vi "HW_Poll_Tracker_1x.vi"(8 "error in":errorcluster, 11 "VISA resource name in":refnum<visa-resource-name>="ASRL3::INSTR") -> (0 "error out":errorcluster, 1 "Read buffer":string, 2 "Parameters output":T1, 3 "VISA resource name out":refnum<visa-resource-name>)   [LabVIEW 2018]
panel:
  out "Sensors response":string
  out "Port data status":i32
  out "Port data status index":i32
  out "FPS status":i32
  out "Poll records":u32
  out "FPS target index":i32
  out "Matrix mode status":string
  out "Matrix mode index":i32
  out "Coordinate mode status":string
  out "Coordinate mode index":i32
  out "Binary mode status":string
  out "Binary mode index":i32
  out "Array of tokens":string[](array[string])
  out "token index":i32
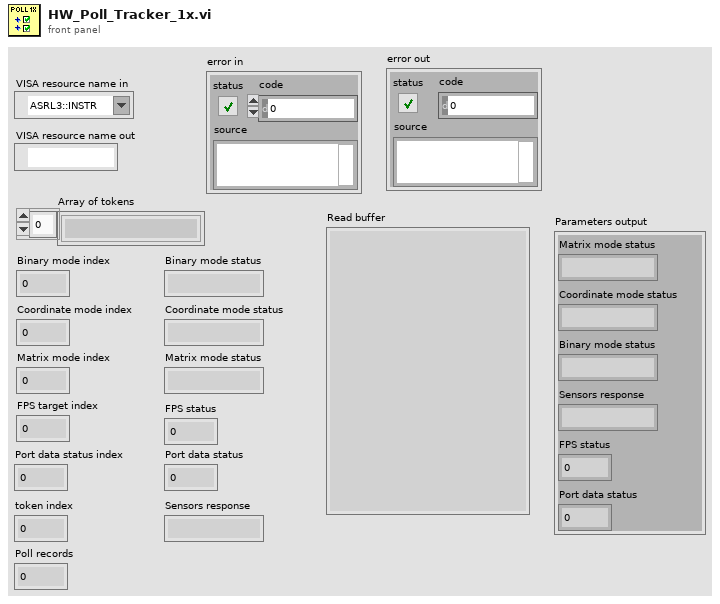
[diagram p1: front panel]
types:
  T1 = cluster{"Matrix mode status":string, "Coordinate mode status":string, "Binary mode status":string, "Sensors response":string, "FPS status":i32, "Port data status":i32}
  T2 = cluster{"token string":string, "token string":string, "token string":string, "trimmed string":string, i32, i32}
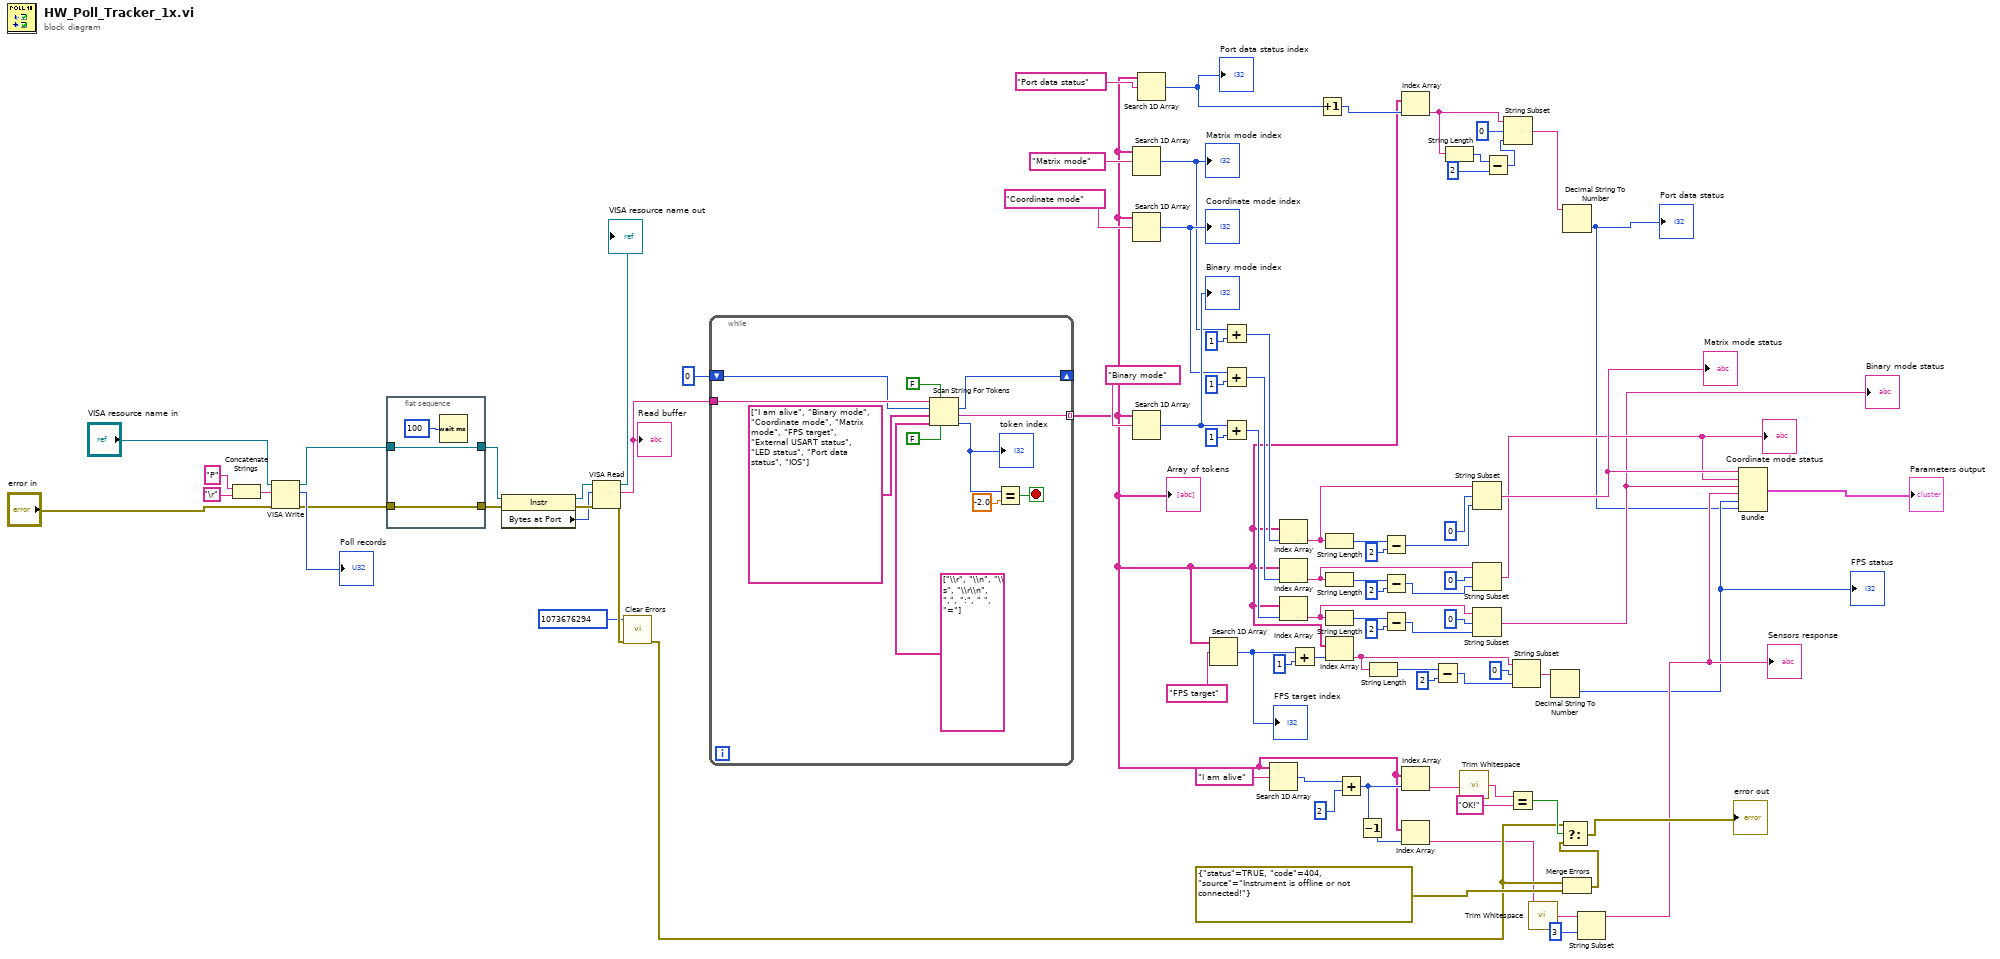
[diagram p0: block diagram]
diagram:
  n1 = Concatenate Strings("P" ("write buffer"), "\r") -> (w86:string)
  n2 = VISA Write(VISA resource name="VISA resource name in", write buffer=w86, error in (no error)="error in") -> (VISA resource name out=w62:refnum<visa-resource-name>, return count=→"Poll records":u32, error out=w60:errorcluster)
  n3 = flat-sequence {
    tunnel: [w90] -> w63
    tunnel: w62 -> [w90]
    tunnel: [w89] -> w61
    tunnel: w60 -> [w89]
    frame #0 {
      n4 = Wait (ms)(milliseconds to wait=u32 100) -> ()  [unwired: 1 out]
    }
  }
  n5 = property class="Instr"(reference=w63, error in=w61) -> (reference out=w84:refnum<visa-resource-name>, error out=w83:errorcluster, "Bytes at Port"=w82:u32)
  n6 = VISA Read(VISA resource name=w84, byte count=w82, error in (no error)=w83) -> (VISA resource name out=→"VISA resource name out":refnum<visa-resource-name>, read buffer=w81:string, error out=w18:errorcluster)  [unwired: 1 out]
  "Read buffer" <- w81
  n7 = call <vilib>:"Clear Errors.vi"("error in (no error)"=w18, "specific error code to clear (0: all)"=1073676294) -> ("error out"=w17:errorcluster)  [unwired: 4 in, 1 out]
  n8 = while {
    tunnel: w81 -> [w102]
    tunnel: [w94] -> w14 mode=indexing
    shift-right: [w93] -> _
    shift-left: 0 ("offset past token") -> [w92]
    stop <- w100 stop-if-true
    n9 = Scan String For Tokens(4:FALSE ("use cached delim/oper data? (F)"), 5:FALSE ("allow empty tokens? (F)"), 6:string[] ["\\r", "\\n", "\\s", "\\r\\n", ",", ":", " ", "="] ("delimiters"), 7:string[] ["I am alive", "Binary mode", "Coordinate mode", "Matrix mode", "FPS target", "External USART status", "LED status", "Port data status", "IOS"] ("Tokens"), 8:w92, 9:w102) -> (0:w98:i32, 1:w94:string, 2:w93:i32)  [unwired: 1 out]
    "token index" <- w98
    n10 = Equal?(x=w98, y=-2.0) -> (x = y?=w100:bool)
  }
  "Array of tokens" <- w14
  n11 = Search 1D Array(1D array=w14, element="Matrix mode") -> (index of element=w70:i32)  [unwired: 1 in]
  "Matrix mode index" <- w70
  n12 = Search 1D Array(1D array=w14, element="Coordinate mode") -> (index of element=w74:i32)  [unwired: 1 in]
  "Coordinate mode index" <- w74
  n13 = Search 1D Array(1D array=w14, element="Binary mode") -> (index of element=w78:i32)  [unwired: 1 in]
  "Binary mode index" <- w78
  n14 = Search 1D Array(1D array=w14, element="Port data status") -> (index of element=w36:i32)  [unwired: 1 in]
  "Port data status index" <- w36
  n15 = Search 1D Array(1D array=w14, element="FPS target") -> (index of element=w66:i32)  [unwired: 1 in]
  "FPS target index" <- w66
  n16 = Add(x=w70, y=1) -> (x+y=w71:i32)
  n17 = Add(x=w74, y=1) -> (x+y=w75:i32)
  n18 = Add(x=w78, y=1) -> (x+y=w79:i32)
  n19 = Search 1D Array(1D array=w14, element="I am alive") -> (index of element=w27:i32)  [unwired: 1 in]
  n20 = Index Array(array=w14, index=w71) -> (element=w40:string)
  n21 = Index Array(array=w14, index=w75) -> (element=w38:string)
  n22 = Index Array(array=w14, index=w79) -> (element=w57:string)
  n23 = Add(x=w66, y=1) -> (x+y=w67:i32)
  n24 = Increment(x=w36) -> (x+1=w35:i32)
  n25 = String Length(string=w40) -> (length=w52:i32)
  n26 = String Length(string=w38) -> (length=w43:i32)
  n27 = String Length(string=w57) -> (length=w56:i32)
  n28 = Index Array(array=w14, index=w67) -> (element=w39:string)
  n29 = Add(x=w27, y=2) -> (x+y=w15:i32)
  n30 = Decrement(x=w15) -> (x-1=w13:i32)
  n31 = String Length(string=w39) -> (length=w48:i32)
  n32 = Subtract(x=w52, y=2) -> (x-y=w50:i32)
  n33 = Subtract(x=w43, y=2) -> (x-y=w41:i32)
  n34 = Subtract(x=w56, y=2) -> (x-y=w54:i32)
  n35 = Index Array(array=w14, index=w35) -> (element=w34:string)
  n36 = Index Array(array=w14, index=w15) -> (element=w25:string)
  n37 = Index Array(array=w14, index=w13) -> (element=w12:string)
  n38 = Subtract(x=w48, y=2) -> (x-y=w46:i32)
  n39 = String Length(string=w34) -> (length=w33:i32)
  n40 = call <vilib>:"Trim Whitespace.vi"("string"=w25) -> ("trimmed string"=w24:string)  [unwired: 1 in]
  n41 = String Subset(string=w40, offset (0)=0, length (rest)=w50) -> (substring=w9:string)
  "Matrix mode status" <- w9
  n42 = String Subset(string=w38, offset (0)=0, length (rest)=w41) -> (substring=w8:string)
  "Coordinate mode status" <- w8
  n43 = String Subset(string=w57, offset (0)=0, length (rest)=w54) -> (substring=w7:string)
  "Binary mode status" <- w7
  n44 = Subtract(x=w33, y=2) -> (x-y=w31:i32)
  n45 = String Subset(string=w34, offset (0)=0, length (rest)=w31) -> (substring=w29:string)
  n46 = Equal?(x=w24, y="OK!") -> (x = y?=w22:bool)
  n47 = String Subset(string=w39, offset (0)=0, length (rest)=w46) -> (substring=w45:string)
  n48 = call <vilib>:"Trim Whitespace.vi"("string"=w12) -> ("trimmed string"=w11:string)  [unwired: 1 in]
  n49 = Decimal String To Number(string=w45) -> (number=w5:i32)  [unwired: 2 in, 1 out]
  "FPS status" <- w5
  n50 = Decimal String To Number(string=w29) -> (number=w4:i32)  [unwired: 2 in, 1 out]
  "Port data status" <- w4
  n51 = Merge Errors(w17, errorcluster {"status"=TRUE, "code"=404, "source"="Instrument is offline or not connected!"} ("error in")) -> (w20:errorcluster)
  n52 = Select(t=w17, s=w22, f=w20) -> (s? t:f=→"error out":errorcluster)
  n53 = String Subset(string=w11, offset (0)=3) -> (substring=w6:string)  [unwired: 1 in]
  "Sensors response" <- w6
  n54 = Bundle("token string"=w9, "token string"=w8, "token string"=w7, "trimmed string"=w6, w5, w4) -> (→"Parameters output":T2)  [unwired: 1 in]
